vi "NI-Embedded CAN for RIO subVI - CAN Frame to Table test.vi"(5 "Boolean":bool, 7 "Hexadecimal?":bool, 8 "x":dbl, 9 "timestamp":timestamp, 10 "Input Array":string[][](array[string]), 11 "CAN frame":T1 {"type" items=["CAN Data", "CAN Remote"]; "identifier" format="%.0x"}) -> (0 "Numeric":dbl, 2 "string":string, 3 "Output Array":string[][](array[string]), 4 "tekst":string, 6 "okres 100":dbl)   [LabVIEW 2015]
doc: "This example shows how to put a CAN transceiver to sleep on RIO Embedded CAN devices."
uses:
  CANFrameControl.ctl
panel:
  out "string 2":string
  out "substring before match":string
  out "subarray 2":string[](array[string])
  out "subarray":string[](array[string])
  in  "Array":T1[](array[typedef]) {"type" items=["CAN Data", "CAN Remote"]; "identifier" format="%.0x"}
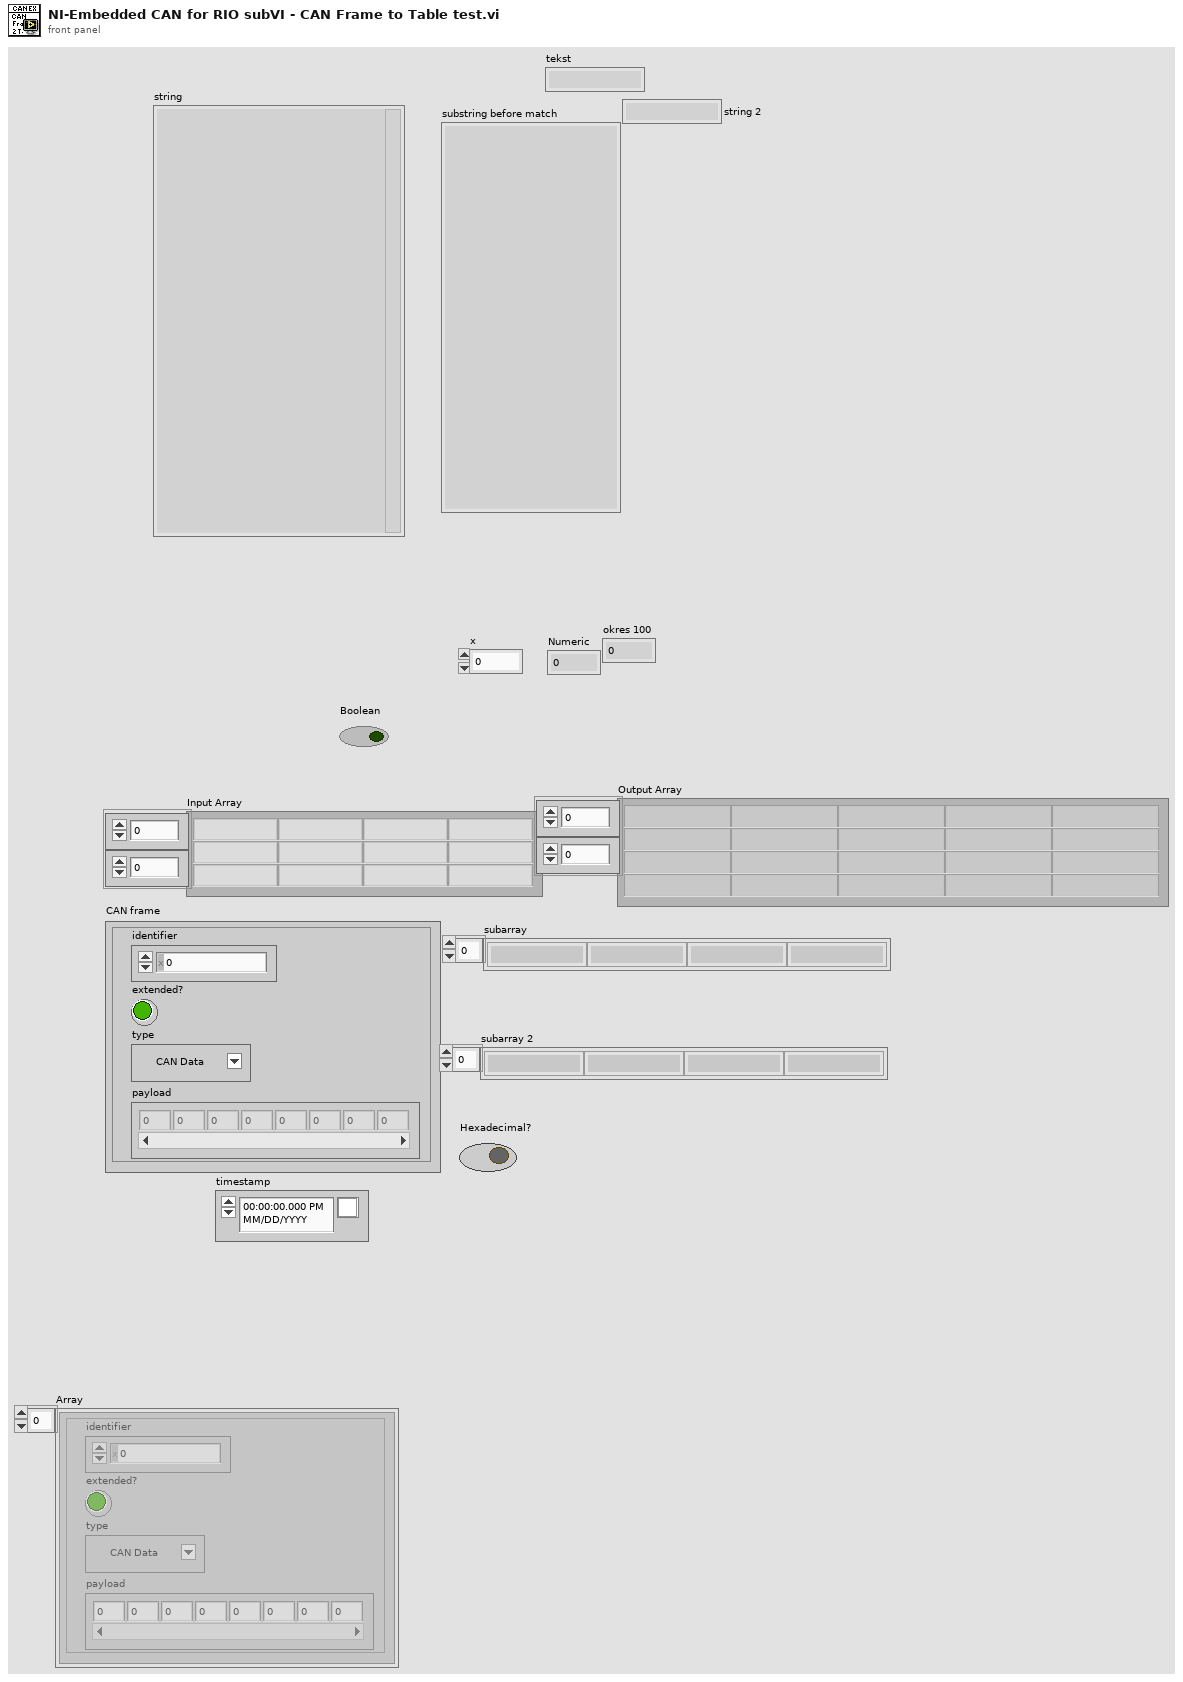
[diagram p1: front panel]
types:
  T1 = typedef "CANFrameControl.ctl" = cluster{"identifier":u32, "extended?":bool, "type":u8, "payload":u8[]}
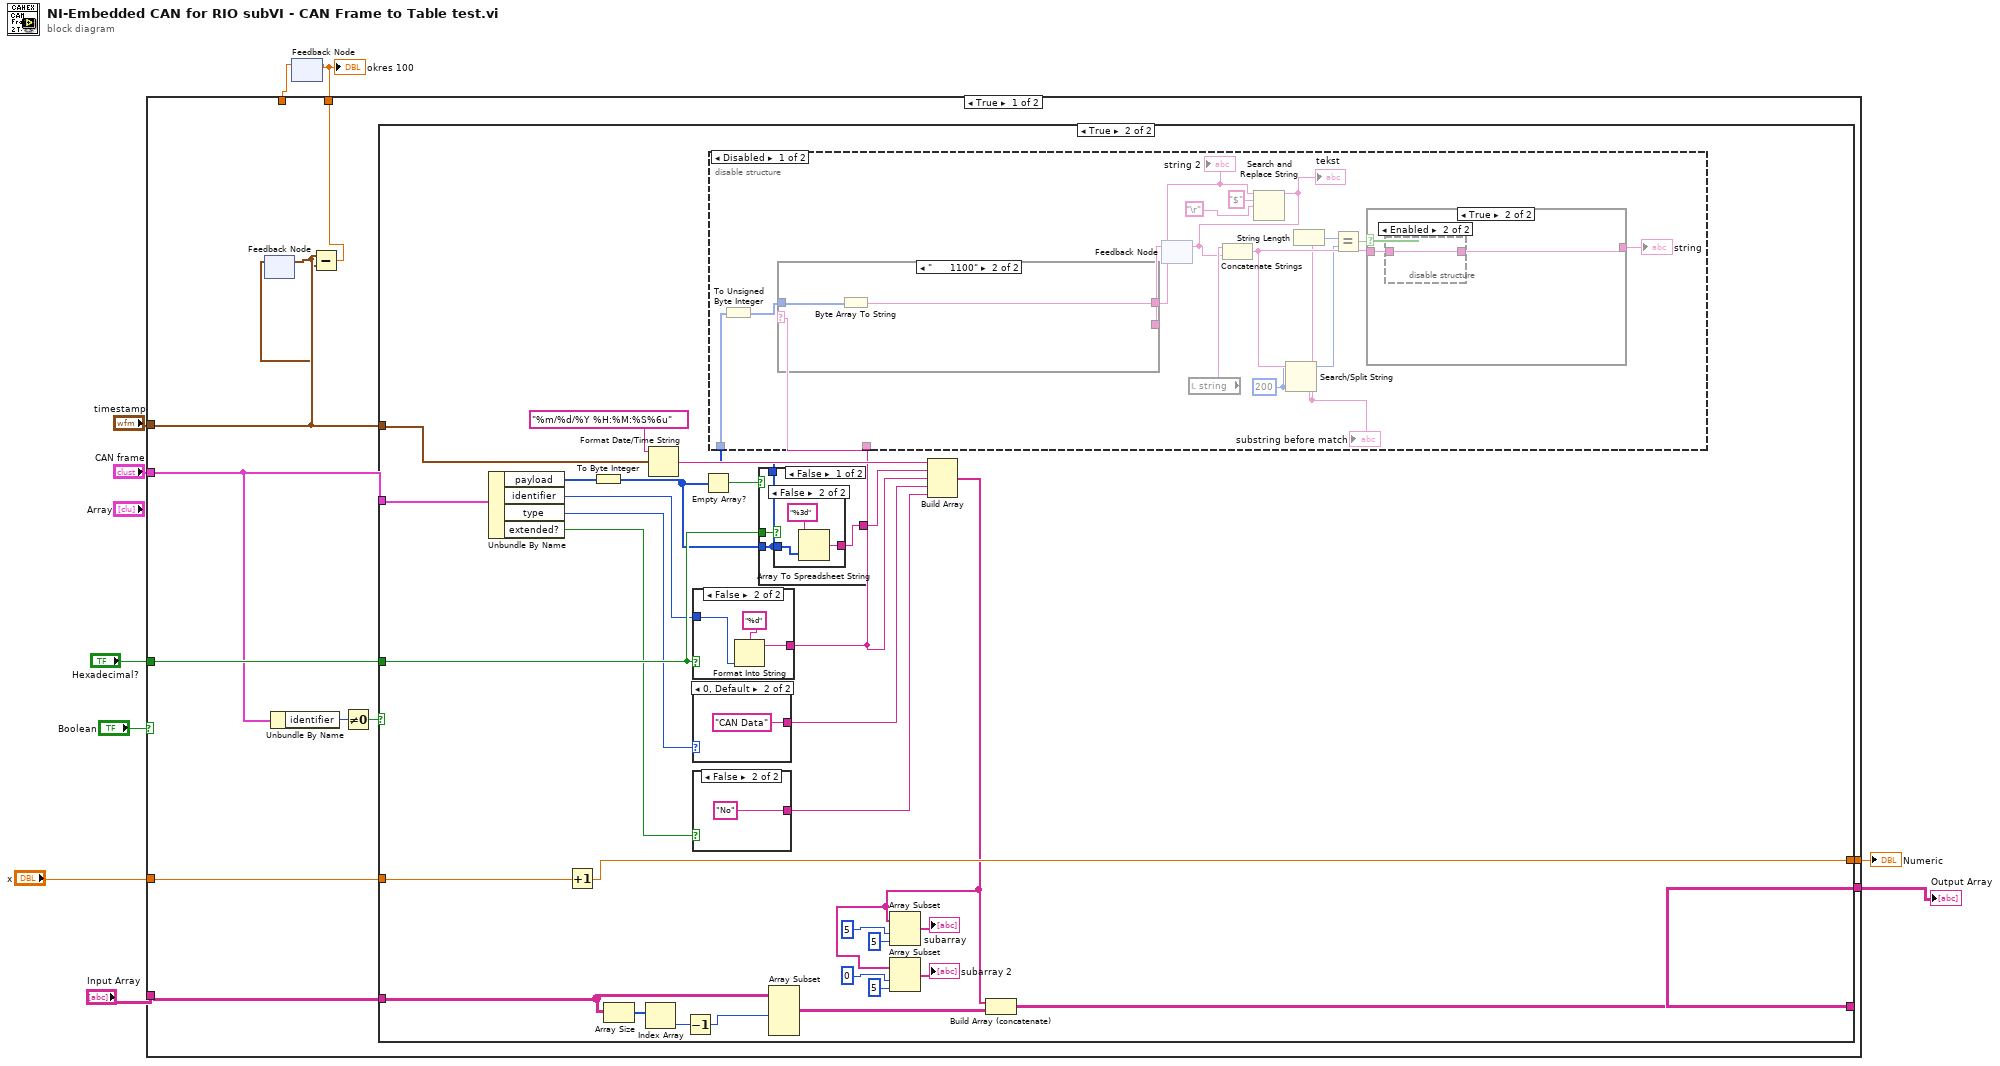
[diagram p0: block diagram]
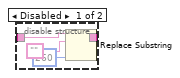
[diagram p4: hidden frame]
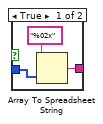
[diagram p7: hidden frame]
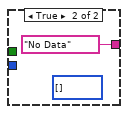
[diagram p8: hidden frame]
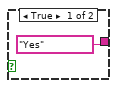
[diagram p9: hidden frame]
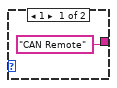
[diagram p10: hidden frame]
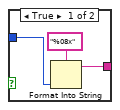
[diagram p11: hidden frame]
diagram:
  n1 = feedback #1() -> (w1:dbl)  [unwired: 1 in]
  n2 = case shown="True" "Boolean" {
    tunnel: "Input Array" -> [w19 w103]
    tunnel: [w21 w103] -> w7
    tunnel: "Hexadecimal?" -> [w20 _]
    tunnel: "CAN frame" -> [w16 _]
    tunnel: "timestamp" -> [w13 _]
    tunnel: [w18 w102] -> w4
    tunnel: "x" -> [w17 w102]
    tunnel: [w14 w101] -> w2
    tunnel: w1 -> [_ w101]
    frame True {
      n3 = feedback #2() -> (w12:timestamp)  [unwired: 1 in]
      n4 = feedback-in #2(w13) -> ()
      n5 = Unbundle By Name(w16) -> ("identifier"=w11:u32)
      n6 = Subtract(x=w13, y=w12) -> (x-y=w14:dbl)
      n7 = Not Equal To 0?(x=w11) -> (x != 0?=w15:bool)
      n8 = case shown="True" w15 {
        tunnel: [w22 w54] -> w21
        tunnel: w20 -> [_ w53]
        tunnel: w13 -> [_ w28]
        tunnel: w19 -> [w22 w52]
        tunnel: w16 -> [_ w51]
        tunnel: [w23 w50] -> w18
        tunnel: w17 -> [w23 w49]
        frame False {
        }
        frame True {
          n9 = Unbundle By Name(w51) -> ("payload"=w25:u8[], "identifier"=w29:u32, "type"=w38:u8, "extended?"=w35:bool)
          n10 = Increment(x=w49) -> (x+1=w50:dbl)
          n11 = To Byte Integer(number=w25) -> (8bit integer=w24:i8[])
          n12 = Array Size(array=w52) -> (size(s)=w48:i32[])
          n13 = Index Array(array=w48) -> (element=w47:i32)  [unwired: 1 in]
          n14 = Format Date/Time String(time format string (%c)="%m/%d/%Y %H:%M:%S%6u", seconds (now)=w28) -> (date/time string=w39:string)  [unwired: 1 in]
          n15 = Decrement(x=w47) -> (x-1=w30:i32)
          n16 = case shown="False" w53 {
            tunnel: w29 -> [w96 w99]
            tunnel: [w95 w98] -> w27
            frame True {
              n17 = Format Into String(format string="%08x", w96) -> (resulting string=w95:string)  [unwired: 2 in, 1 out]
            }
            frame False {
              n18 = Format Into String(format string="%d", w99) -> (resulting string=w98:string)  [unwired: 2 in, 1 out]
            }
          }
          n19 = case shown="0, Default" w38 {
            tunnel: ["CAN Remote" "CAN Data"] -> w37
            frame 1 {
            }
            frame 0, Default {
            }
          }
          n20 = case shown="False" w35 {
            tunnel: ["Yes" "No"] -> w36
            frame True {
            }
            frame False {
            }
          }
          n21 = Empty Array?(array=w24) -> (empty?=w32:bool)
          n22 = case shown="False" w32 {
            tunnel: [w82 "No Data"] -> w34
            tunnel: w24 -> [w81 _]
            tunnel: w53 -> [w83 _]
            tunnel: [w81 _] -> w26
            frame False {
              n23 = case shown="False" w83 {
                tunnel: w81 -> [w84 w87]
                tunnel: [w85 w88] -> w82
                frame True {
                  n24 = Array To Spreadsheet String(array=w84, 3:"%02x" ("format string")) -> (spreadsheet string=w85:string)  [unwired: 1 in]
                }
                frame False {
                  n25 = Array To Spreadsheet String(array=w87, 3:"%3d" ("format string")) -> (spreadsheet string=w88:string)  [unwired: 1 in]
                }
              }
            }
            frame True {
              (unwired) u8[] [] ("payload")
            }
          }
          n26 = disable-structure shown="Disabled" {
            disable-tunnel: w27 -> [w69 _]
            disable-tunnel: w26 -> [w55 _]
            frame Disabled {
              w57 = 200 ("offset (0)")
              n27 = To Unsigned Byte Integer(number=w55) -> (unsigned 8bit integer=w56:u8[])
              n28 = feedback #3() -> (w68:string)  [unwired: 1 in]
              n29 = case shown="\"      1100\"" w69 {
                tunnel: w56 -> [_ w80]
                tunnel: [w78 w79] -> w65
                tunnel: w68 -> [w78 _]
                frame "False", Default {
                }
                frame "      1100" {
                  n30 = Byte Array To String(unsigned byte array=w80) -> (string=w79:string)
                }
              }
              "string 2" <- w65
              n31 = local read "string"() -> (w63:string)
              n32 = Search and Replace String(input string=w65, search string="$", replace string="\r") -> (result string=w61:string)  [unwired: 5 in, 3 out]
              "tekst" <- w61
              n33 = feedback-in #3(w61) -> ()
              n34 = Concatenate Strings(w63, w61) -> (w62:string)
              n35 = Search/Split String(string=w62, offset (0)=w57) -> (substring before match=w58:string)  [unwired: 1 in, 2 out]
              "substring before match" <- w58
              n36 = String Length(string=w58) -> (length=w60:i32)
              n37 = Equal?(x=w60, y=w57) -> (x = y?=w59:bool)
              n38 = case shown="True" w59 {
                tunnel: [w70 w72] -> w64
                tunnel: w62 -> [w70 w71]
                frame False {
                }
                frame True {
                  n39 = disable-structure shown="Enabled" {
                    disable-tunnel: [w76 w77] -> w72
                    disable-tunnel: w71 -> [w75 w77]
                    frame Disabled {
                      n40 = Replace Substring(2:260 ("length (len. of substring)"), 4:"", 5:w75) -> (1:w76:string)  [unwired: 1 in, 1 out]
                    }
                    frame Enabled {
                    }
                  }
                }
              }
              "string" <- w64
            }
            frame Enabled {
            }
          }
          n41 = Array Subset(array=w52, length (row)=w30) -> (w40:string[][])  [unwired: 3 in]
          n42 = Build Array(w39, w34, w27, w37, w36) -> (w31:string[])
          n43 = Array Subset(array=w31, index=5 ("length"), length=5) -> (→"subarray":string[])
          n44 = Array Subset(array=w31, index=0 ("length"), length=5) -> (→"subarray 2":string[])
          n45 = Build Array (concatenate)(w31, w40) -> (w54:string[][])
        }
      }
    }
    frame False {
    }
  }
  "Output Array" <- w7
  "Numeric" <- w4
  "okres 100" <- w2
  n46 = feedback-in #1(w2) -> ()
